vi "RunTest.vi"(8 "error in (no error)":errorcluster, 11 "Prueba02 in":refnum<class "Prueba02.lvclass">) -> (0 "error out":errorcluster, 2 "resultado":string, 3 "Prueba02 out":refnum<class "Prueba02.lvclass">)   [LabVIEW 2019, in "Prueba02.lvclass"]
uses:
  Prueba02.lvclass
  Prueba02.lvclass/Prueba02.ctl
panel:
  out "cumple_no cumple":bool
  out "Pict Ring 2":u16(ring)
  out "Pict Ring":u16(ring)
  in  "Tabla":string[][](table)
  in  "seguir":bool
  out "no_cumple":bool
  out "cumple":bool
  # "Cumple"
  # "No Cumple"
  # "2. Ruido Intrínseco. IEC 61672-3: 2006 Cláusula 10"
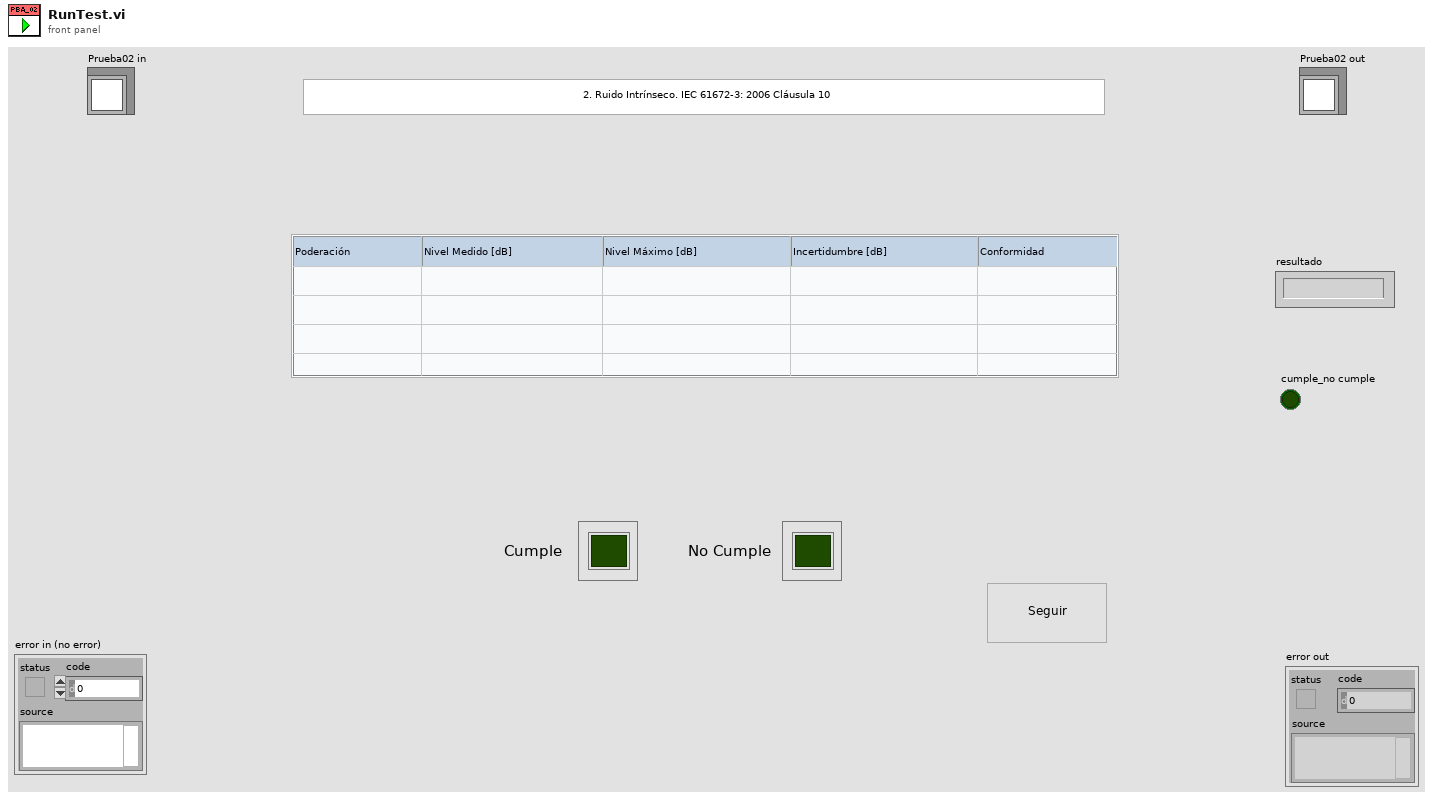
[diagram p1: front panel]
types:
  T1 = typedef "LVRowAndColumnTypeDef.ctl" = cluster{"Row":i32, "Column":i32}
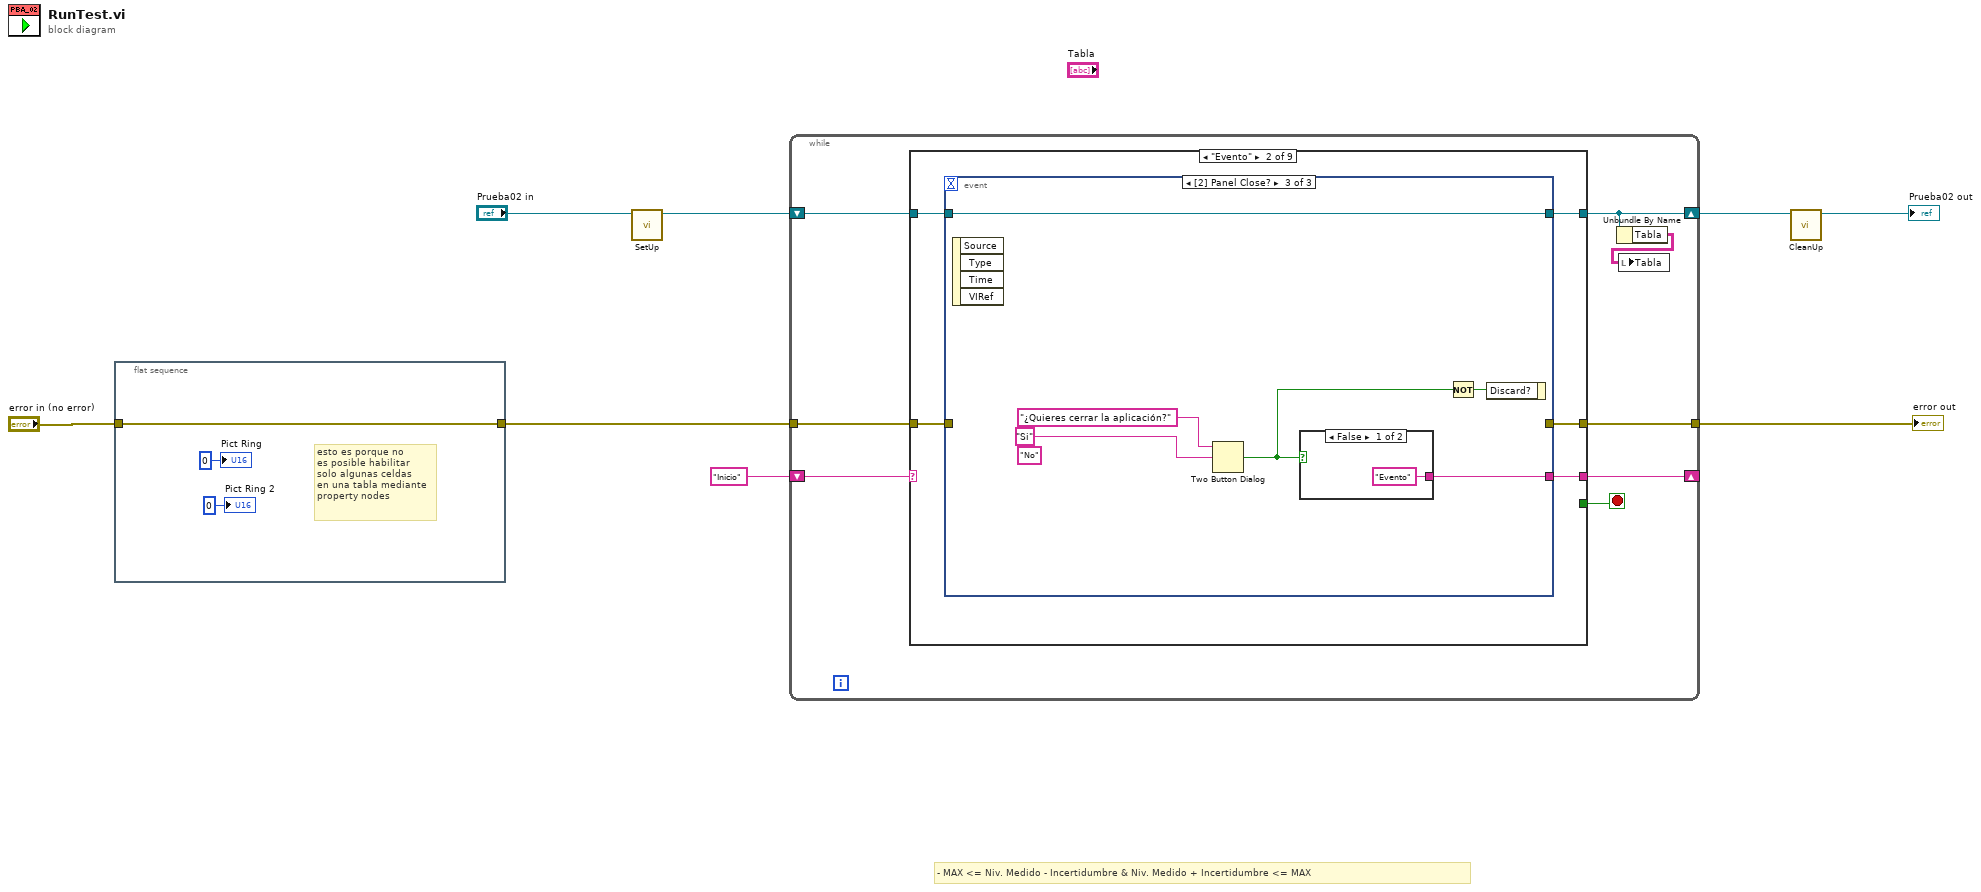
[diagram p0: block diagram]
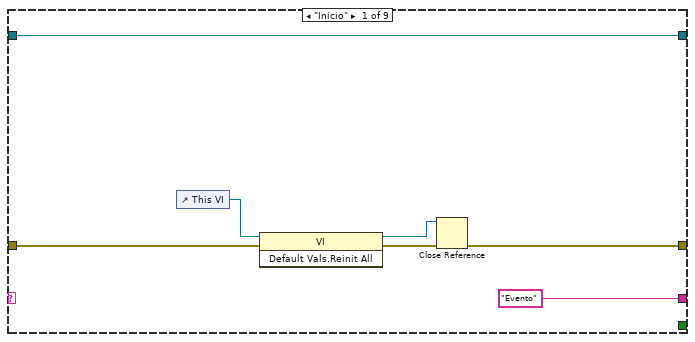
[diagram p2: hidden frame]
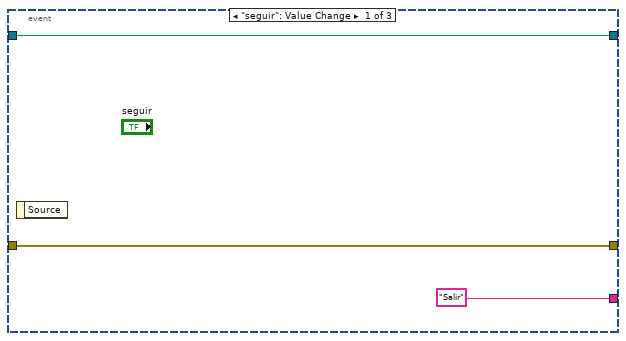
[diagram p3: hidden frame]
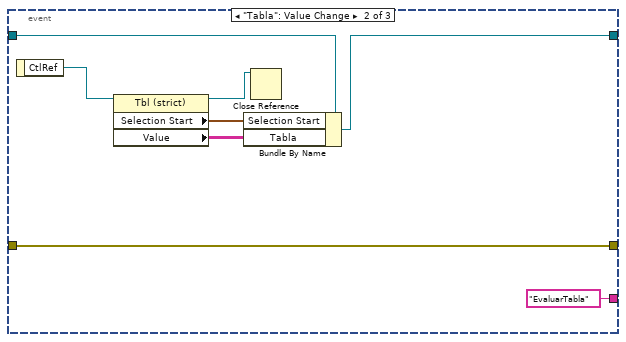
[diagram p4: hidden frame]
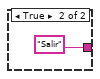
[diagram p5: hidden frame]
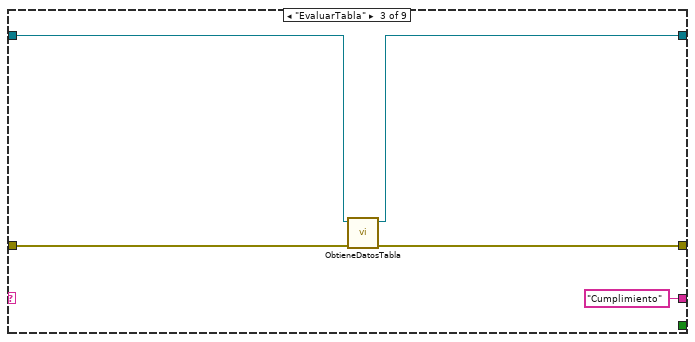
[diagram p6: hidden frame]
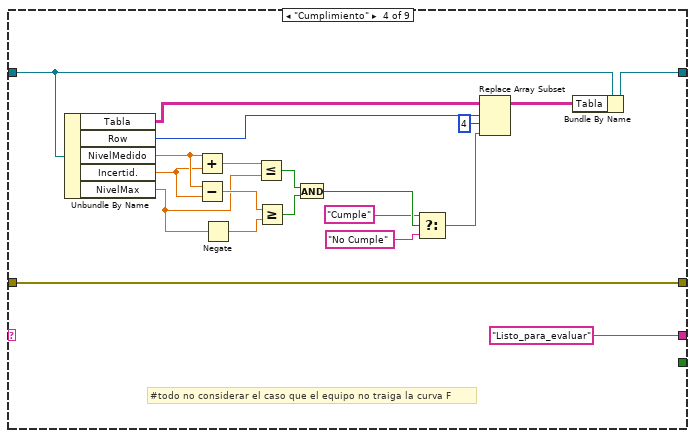
[diagram p7: hidden frame]
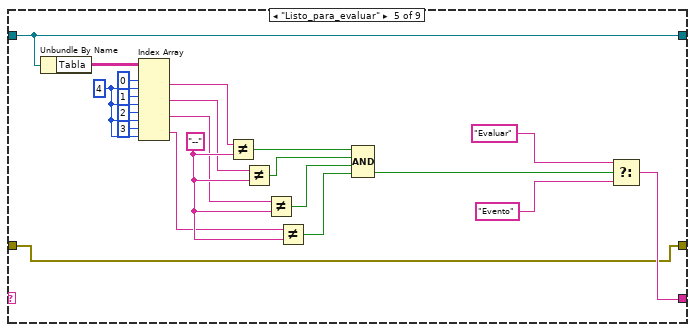
[diagram p8: hidden frame]
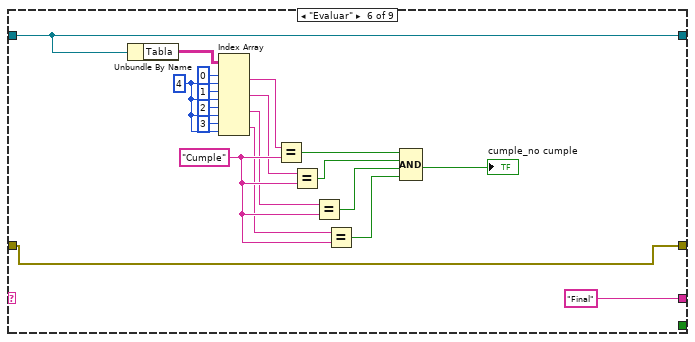
[diagram p9: hidden frame]
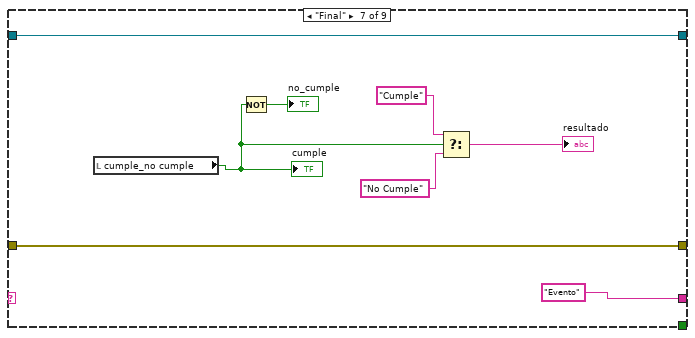
[diagram p10: hidden frame]
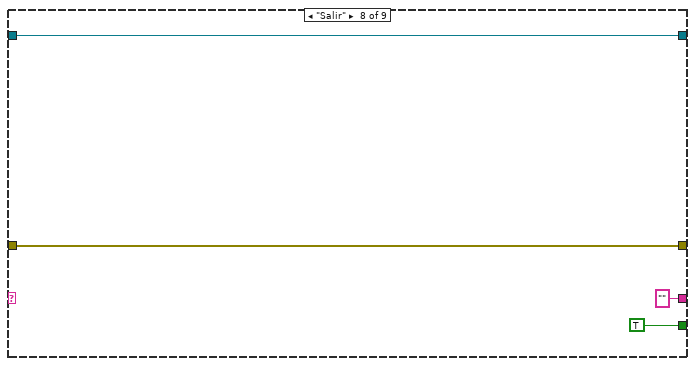
[diagram p11: hidden frame]
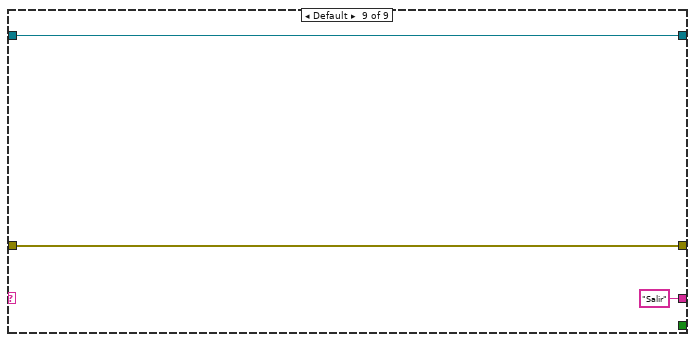
[diagram p12: hidden frame]
diagram:
  # "- MAX <= Niv. Medido - Incertidumbre & Niv. Medido + Incertidumbre <= MAX"
  n1 = flat-sequence {
    tunnel: [w9] -> w3
    tunnel: "error in (no error)" -> [w9]
    frame #0 {
      # "esto es porque no\nes posible habilitar\nsolo algunas celdas\nen una tabla mediante\nproperty nodes"
      "Pict Ring" <- u16 0 ("Pict Ring")
      "Pict Ring 2" <- u16 0 ("Pict Ring 2")
    }
  }
  n2 = call-dynamic "SetUp.vi"("Prueba02 in"="Prueba02 in") -> ("Prueba02 out"=w5:refnum<class "Prueba02.lvclass">)  [unwired: 9 in, 1 out]
  n3 = while {
    shift-right: [w18] -> _
    shift-left: "Inicio" -> [w19]
    tunnel: w3 -> [w15]
    shift-right: [w17] -> w6
    shift-left: w5 -> [w13]
    tunnel: [w14] -> w4
    stop <- w12 stop-if-true
    n4 = case shown="\"Evento\"" w19 {
      tunnel: ["Evento" w31 "Cumplimiento" "Listo_para_evaluar" w84 "Final" "Evento" "" "Salir"] -> w18
      tunnel: w13 -> [w22 w30 w53 w65 w81 w102 w117 w127 w128]
      tunnel: [w22 w29 w52 w58 w81 w102 w117 w127 w128] -> w17
      tunnel: w15 -> [w21 w27 w55 w59 w82 w103 w116 w126 w130]
      tunnel: [w20 w28 w54 w59 w82 w103 w116 w126 w130] -> w14
      tunnel: [_ _ _ _ _ _ _ TRUE _] -> w12
      frame "Inicio" {
        n5 = control-ref of="This VI"() -> (w23:refnum<vi>)
        n6 = invoke class="VI" method="Default Vals.Reinit All"(reference=w23, error in=w21) -> (reference out=w24:refnum<vi>, error out=w25:errorcluster)  [unwired: 1 in, 1 out]
        n7 = Close Reference(reference=w24, error in (no error)=w25) -> (error out=w20:errorcluster)
      }
      frame "Evento" {
        n8 = event shown="[2] Panel Close?" {
          selector: _ -> [_ _ _]
          dyn-events: _ -> [_ _ _]
          timeout: _ -> [_ _ _]
          tunnel: ["Salir" "EvaluarTabla" w46] -> w31
          tunnel: w30 -> [w34 w40 w43]
          tunnel: [w34 w39 w43] -> w29
          tunnel: [w33 w41 _] -> w28
          tunnel: w27 -> [w33 w41 _]
          event "seguir": Value Change {
            n9 = event-data() -> ()  [unwired: 1 in, 1 out]
          }
          event "Tabla": Value Change {
            n10 = event-data() -> ("CtlRef"=w38:refnum<vi>)  [unwired: 1 in]
            n11 = property class="Tbl (strict)"(reference=w38) -> (reference out=w35:refnum<vi>, "Selection Start"=w37:T1, "Value"=w36:string[][])  [unwired: 1 in, 1 out]
            n12 = Bundle By Name(cluster=w40, "Selection Start"=w37, "Tabla"=w36) -> (w39:refnum<class "Prueba02.lvclass">)
            n13 = Close Reference(reference=w35) -> ()  [unwired: 1 in, 1 out]
          }
          event Panel Close? {
            (unwired) "No" ("T button name (\"OK\")")
            n14 = event-data() -> ()  [unwired: 1 in, 4 out]
            n15 = Two Button Dialog(message="¿Quieres cerrar la aplicación?", 2:"Si" ("T button name (\"OK\")")) -> (T button?=w44:bool)  [unwired: 1 in]
            n16 = case shown="False" w44 {
              tunnel: ["Evento" "Salir"] -> w46
              frame False {
              }
              frame True {
              }
            }
            n17 = Not(x=w44) -> (.not. x?=w45:bool)
            n18 = event-data("Discard?"=w45) -> ()  [unwired: 1 in, 1 out]
          }
        }
      }
      frame "EvaluarTabla" {
        n19 = call "ObtieneDatosTabla.vi"("error in (no error)"=w55, "Prueba02 in"=w53) -> ("error out"=w54:errorcluster, "Prueba02 out"=w52:refnum<class "Prueba02.lvclass">)  [unwired: 8 in]
      }
      frame "Cumplimiento" {
        # "#todo no considerar el caso que el equipo no traiga la curva F"
        n20 = Unbundle By Name(w65) -> ("Tabla"=w56:string[][], "Row"=w64:i32, "NivelMedido"=w62:dbl, "Incertid."=w61:dbl, "NivelMax"=w60:dbl)
        n21 = Add(x=w62, y=w61) -> (x+y=w74:dbl)
        n22 = Subtract(x=w62, y=w61) -> (x-y=w71:dbl)
        n23 = Negate(x=w60) -> (-x=w70:dbl)
        n24 = Less Or Equal?(x=w74, y=w60) -> (x <= y?=w73:bool)
        n25 = Greater Or Equal?(x=w71, y=w70) -> (x >= y?=w72:bool)
        n26 = And(x=w73, y=w72) -> (x .and. y?=w69:bool)
        n27 = Select(t="Cumple", s=w69, f="No Cumple") -> (s? t:f=w66:string)
        n28 = Replace Array Subset(array=w56, new element=w66, index (row)=w64, index (col)=4 ("disabled index (col)")) -> (w57:string[][])
        n29 = Bundle By Name(cluster=w65, "Tabla"=w57) -> (w58:refnum<class "Prueba02.lvclass">)
      }
      frame "Listo_para_evaluar" {
        w91 = "--" ("y")
        w96 = 4 ("disabled index (col)")
        n30 = Unbundle By Name(w81) -> ("Tabla"=w80:string[][])
        n31 = Index Array(array=w80, index (row) #1=0 ("disabled index (row)"), index (col) #1=w96, index (row) #2=1 ("disabled index (row)"), index (col) #2=w96, index (row) #3=2 ("disabled index (row)"), index (col) #3=w96, index (row) #4=3 ("disabled index (row)"), index (col) #4=w96) -> (element #1=w79:string, element #2=w78:string, element #3=w77:string, element #4=w76:string)
        n32 = Not Equal?(x=w79, y=w91) -> (x != y?=w90:bool)
        n33 = Not Equal?(x=w78, y=w91) -> (x != y?=w89:bool)
        n34 = Not Equal?(x=w77, y=w91) -> (x != y?=w88:bool)
        n35 = Not Equal?(x=w76, y=w91) -> (x != y?=w87:bool)
        n36 = Compound Arithmetic op=AND(w90, w89, w88, w87) -> (w83:bool)
        n37 = Select(t="Evaluar", s=w83, f="Evento") -> (s? t:f=w84:string)
      }
      frame "Evaluar" {
        w110 = "Cumple" ("y")
        w115 = 4 ("disabled index (col)")
        n38 = Unbundle By Name(w102) -> ("Tabla"=w101:string[][])
        n39 = Index Array(array=w101, index (row) #1=0 ("disabled index (row)"), index (col) #1=w115, index (row) #2=1 ("disabled index (row)"), index (col) #2=w115, index (row) #3=2 ("disabled index (row)"), index (col) #3=w115, index (row) #4=3 ("disabled index (row)"), index (col) #4=w115) -> (element #1=w100:string, element #2=w99:string, element #3=w98:string, element #4=w97:string)
        n40 = Equal?(x=w100, y=w110) -> (x = y?=w109:bool)
        n41 = Equal?(x=w99, y=w110) -> (x = y?=w108:bool)
        n42 = Equal?(x=w98, y=w110) -> (x = y?=w107:bool)
        n43 = Equal?(x=w97, y=w110) -> (x = y?=w106:bool)
        n44 = Compound Arithmetic op=AND(w109, w108, w107, w106) -> (→"cumple_no cumple":bool)
      }
      frame "Final" {
        n45 = local read "cumple_no cumple"() -> (w118:bool)
        "cumple" <- w118
        n46 = Not(x=w118) -> (.not. x?=→"no_cumple":bool)
        n47 = Select(t="Cumple", s=w118, f="No Cumple") -> (s? t:f=→"resultado":string)
      }
      frame "Salir" {
      }
      frame Default {
      }
    }
    n48 = Unbundle By Name(w17) -> ("Tabla"=w16:string[][])
    n49 = local write "Tabla"(w16) -> ()
  }
  "error out" <- w4
  n50 = call-dynamic "CleanUp.vi"("Prueba02 in"=w6) -> ("Prueba02 out"=→"Prueba02 out":refnum<class "Prueba02.lvclass">)  [unwired: 9 in, 1 out]
